vi "GFITS_GetLocalValues.vi"(6 "Types":T1={"TBIT"=1, "TBYTE"=11, "TSTRING"=16, "TSHORT"=21, "TLONG"=41, "TFLOAT"=42, "TDOUBLE"=82, "TCOMPLEX"=83, "TDBLCOMPLEX"=163, "TUINT"=30, "TUSHORT"=20, "TULONG"=40, "TINT"=31, "TSBYTE"=12, "TLONGLONG"=81, "TLOGICAL"=14}, 8 "error in (no error)":errorcluster, 10 "key":string) -> (0 "error out":errorcluster, 1 "datatype":u16, 2 "value":string)   [LabVIEW 2016]
uses:
  GFITS_datatypesctl.ctl
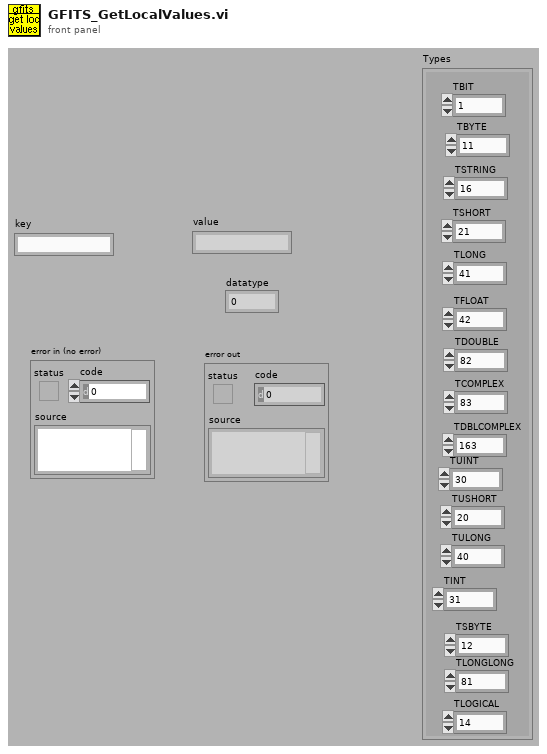
[diagram p1: front panel]
types:
  T1 = typedef "GFITS_datatypesctl.ctl" = cluster{"TBIT":i32, "TBYTE":i32, "TSTRING":i32, "TSHORT":i32, "TLONG":i32, "TFLOAT":i32, "TDOUBLE":i32, "TCOMPLEX":i32, "TDBLCOMPLEX":i32, "TUINT":i32, "TUSHORT":i32, "TULONG":i32, "TINT":i32, "TSBYTE":i32, "TLONGLONG":i32, "TLOGICAL":i32}
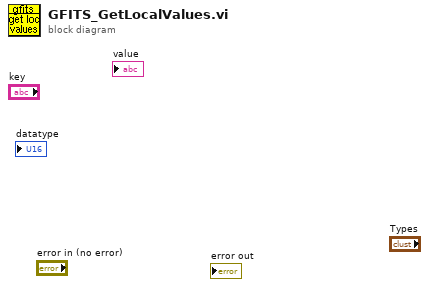
[diagram p0: block diagram]
diagram:
